vi "Try Get Object Entry.vi"(8 "error in":errorcluster, 10 "Index":u16 format="%04x", 11 "Object Dictionary in":refnum<class "Object Dictionary.lvclass">) -> (0 "error out":errorcluster, 1 "Object Entry":refnum<class "Object Entry.lvclass">, 2 "Success":bool, 3 "Object Dictionary out":refnum<class "Object Dictionary.lvclass">)   [LabVIEW 2020, in "CANopen.lvlib" / "Object Dictionary.lvclass"]
doc: "When this method returns, contains the value associated with the specified key, if the key is found; otherwise, the default value for the type of the value parameter. This parameter is passed uninitialized."
uses:
  Object Dictionary.lvclass
  Object Entry/Object Entry.lvclass
  Object Dictionary.lvclass/Object Dictionary.ctl
  Ordered-Dictionary/Ordered Object Dictionary/Source/Ordered Object Dictionary.lvclass
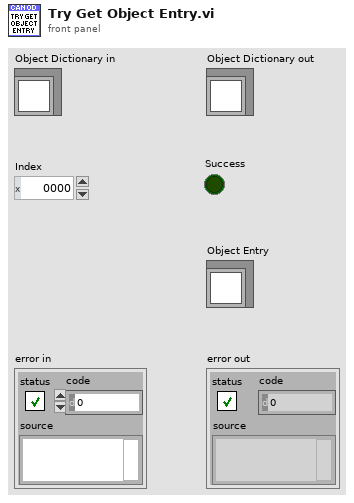
[diagram p1: front panel]
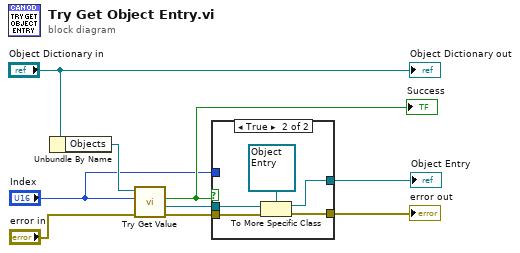
[diagram p0: block diagram]
diagram:
  n1 = Unbundle By Name("Object Dictionary in") -> ("Objects"=w4:refnum<class "Ordered Object Dictionary.lvclass">)
  n2 = call "Try Get Value.vi"("error in"="error in", "Key"="Index", "Ordered Object Dictionary in"=w4) -> ("error out"=w9:errorcluster, "Value"=w3:refnum<class>, "Success"=w2:bool)  [unwired: 5 in, 1 out]
  "Success" <- w2
  n3 = case shown="True" w2 {
    tunnel: w9 -> [w10 w15]
    tunnel: [w10 w14] -> w8
    tunnel: w3 -> [_ w13]
    tunnel: [_ w12] -> w7
    tunnel: "Index" -> [_ _]
    frame False {
    }
    frame True {
      n4 = To More Specific Class(target class=refnum<class "Object Entry.lvclass"> refnum ("CANopen.lvlib:Obj Entry"), reference=w13, error in=w15) -> (specific class reference=w12:refnum<class "Object Entry.lvclass">, error out=w14:errorcluster)
    }
  }
  "error out" <- w8
  "Object Entry" <- w7
  "Object Dictionary out" <- "Object Dictionary in"
